vi "Test Write Read Class.vi"(11 "Test Case In":refnum<class "Singleton.lvclass">) -> (0 "error out":errorcluster, 3 "Test Case Out":refnum<class "Singleton.lvclass">)   [LabVIEW 2020, in "Singleton.lvclass"]
uses:
  Singleton.lvclass
  C:/Program Files (x86)/National Instruments/LabVIEW 2020/vi.lib/Astemes/LUnit/Test Case.lvclass
  Basic Class/Basic Class.lvclass
  Basic Class/Basic Class.lvclass/Basic Class.ctl
  <vilib>/Astemes/LUnit/Test Case.lvclass/Test Case.ctl
  4993e8ee-a06a-463a-9684-69129f64d5ce.vi
  <vilib>/Astemes/LUnit/Core/LUnit Test Case/Private/Append Pass Result.vi
  <vilib>/Astemes/LUnit/Core/LUnit Test Case/Private/Append Fail Result.vi
  4993e8ee-a06a-463a-9684-69129f64d5ce.vi/9c5d11cd-9439-4240-a1ee-d9baace9c924.vi
  <vilib>/Astemes/LUnit/Core/LUnit Test Case/Private/Run In UI.vi
  <vilib>/Utility/error.llb/Clear Errors.vi
  Singleton.lvclass/Singleton.ctl
  Source/Provider/Provider.lvclass
  <vilib>/Astemes/LUnit/Test Case.lvclass
  C:/Program Files (x86)/National Instruments/LabVIEW 2020/vi.lib/Astemes/LUnit/LUnit Runnable.lvclass
  C:/Users/hughe_cx/Documents/05_repos/LVLog/Testing/Singleton/Singleton.lvclass
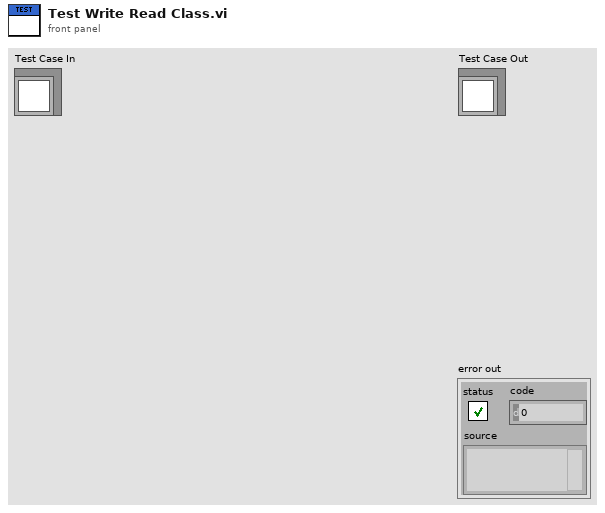
[diagram p1: front panel]
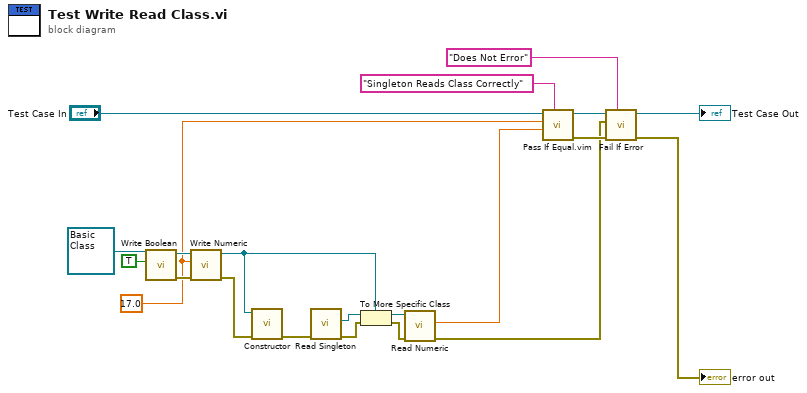
[diagram p0: block diagram]
diagram:
  w9 = 17.0 ("Numeric")
  n1 = call "Write Boolean.vi"("Boolean"=TRUE, "Basic Class in"=refnum<class "Basic Class.lvclass"> refnum ("Basic Class.lvclass")) -> ("error out"=w18:errorcluster, "Basic Class out"=w19:refnum<class "Basic Class.lvclass">)  [unwired: 8 in]
  n2 = call "Write Numeric.vi"("error in (no error)"=w18, "Numeric"=w9, "Basic Class in"=w19) -> ("error out"=w17:errorcluster, "Basic Class out"=w13:refnum<class "Basic Class.lvclass">)  [unwired: 7 in]
  n3 = call "Constructor.vi"("error in (no error)"=w17, "Class in"=w13) -> ("error out"=w20:errorcluster)  [unwired: 8 in, 1 out]
  n4 = call "Read Singleton.vi"("error in (no error)"=w20) -> ("error out"=w14:errorcluster, "Object Data Out"=w12:refnum<class>)  [unwired: 9 in]
  n5 = To More Specific Class(target class=w13, reference=w12, error in=w14) -> (specific class reference=w11:refnum<class "Basic Class.lvclass">, error out=w7:errorcluster)
  n6 = call "Read Numeric.vi"("error in (no error)"=w7, "Basic Class in"=w11) -> ("error out"=w2:errorcluster, "Numeric"=w10:dbl)  [unwired: 7 in, 1 out]
  n7 = call "Pass If Equal.vim"("Description"="Singleton Reads Class Correctly", "Actual"=w10, "Expected"=w9, "LUnit Test Case In"="Test Case In") -> ("error out"=w5:errorcluster, "LUnit Test Case Out"=w6:refnum<class "Singleton.lvclass">)  [unwired: 6 in]
  n8 = call <vilib>:"Fail If Error.vi"("Description"="Does Not Error", "error in (no error)"=w5, "Assert error"=w2, "LUnit Test Case In"=w6) -> ("error out"=→"error out":errorcluster, "LUnit Test Case Out"=→"Test Case Out":refnum<class "Singleton.lvclass">)  [unwired: 6 in]
